vi "Look Ahead Distance (SubVI).vi"(1 "velocity(kph)":dbl) -> (0 "ld(m)":dbl)   [LabVIEW 2015]
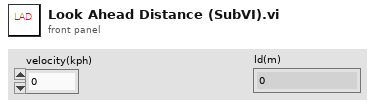
[diagram p1: front panel]
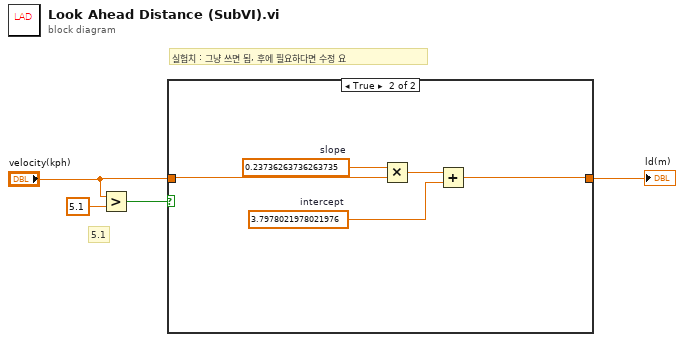
[diagram p0: block diagram]
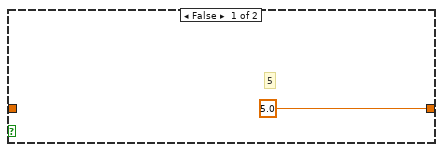
[diagram p2: hidden frame]
diagram:
  # "실험치 : 그냥 쓰면 됨, 후에 필요하다면 수정 요"
  # "5.1"
  n1 = Greater?(x="velocity(kph)", y=5.1) -> (0:w2:bool)
  n2 = case shown="True" w2 {
    tunnel: "velocity(kph)" -> [_ w7]
    tunnel: [5.0 w6] -> w1
    frame False {
      # "5"
    }
    frame True {
      w8 = 3.7978021978021976  # intercept
      w10 = 0.23736263736263735  # slope
      n3 = Multiply(x=w10, y=w7) -> (x*y=w9:dbl)
      n4 = Add(x=w9, y=w8) -> (x+y=w6:dbl)
    }
  }
  "ld(m)" <- w1
